vi "Sub_FEA_Make_M_and K_Matrices_online.vi"(10 "FEA matrices":cluster{"Mass":dbl[][], "Stiffness":dbl[][]}, 11 "Pin Location":i32) -> (2 "Mass":dbl[][](array[numeric]), 3 "Stiff":dbl[][](array[numeric]))   [LabVIEW 2019]
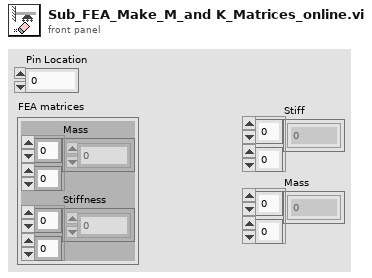
[diagram p1: front panel]
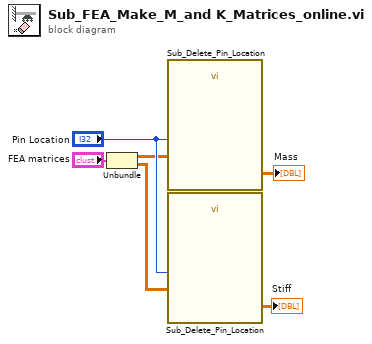
[diagram p0: block diagram]
diagram:
  n1 = Unbundle("FEA matrices") -> ("Mass"=w2:dbl[][], "Stiffness"=w1:dbl[][])
  n2 = call "Sub_Delete_Pin_Location.vi"("Pre-Pin Matrix"=w2, "Pin Location"="Pin Location") -> ("Post-Pin Matrix"=→"Mass":dbl[][])  [unwired: 9 in]
  n3 = call "Sub_Delete_Pin_Location.vi"("Pre-Pin Matrix"=w1, "Pin Location"="Pin Location") -> ("Post-Pin Matrix"=→"Stiff":dbl[][])  [unwired: 9 in]
